vi "DAQ Process.vi"(10 "DAQ Process UE Refnum":T1, 11 "All Stop":refnum<user-event>) -> ()   [LabVIEW 2011]
doc: "Continuously generates Data and Error user events for the DAQ Process."
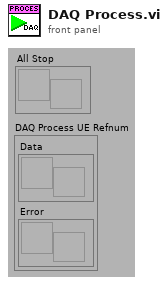
[diagram p1: front panel]
types:
  T1 = cluster{"Data":refnum<user-event>, "Error":refnum<user-event>}
  T2 = cluster{"seconds since 1Jan1904":timestamp, i32, dbl[]}
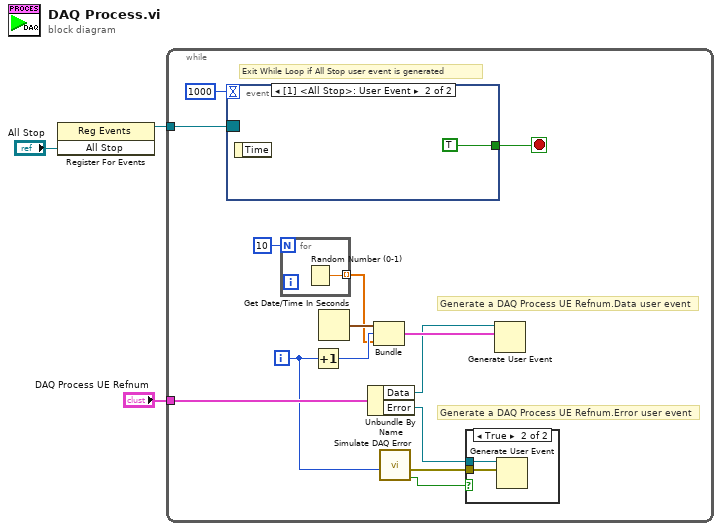
[diagram p0: block diagram]
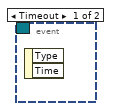
[diagram p3: hidden frame]
diagram:
  n1 = register-events("All Stop") -> (reference out=w2:refnum<event-registration>)  [unwired: 2 in, 1 out]
  n2 = while {
    tunnel: w2 -> [w15]
    tunnel: "DAQ Process UE Refnum" -> [w13]
    i -> [w8]
    stop <- w16 stop-if-true
    # "Generate a DAQ Process UE Refnum.Error user event"
    # "Generate a DAQ Process UE Refnum.Data user event"
    # "Exit While Loop if All Stop user event is generated"
    n3 = event shown="[1] <All Stop>: User Event" {
      selector: w15 -> [_ _]
      dyn-events: _ -> [_ _]
      timeout: 1000 -> [_ _]
      tunnel: [_ TRUE] -> w16
      event Timeout {
        n4 = event-data() -> ()  [unwired: 1 in, 2 out]
      }
      event User Event {
        n5 = event-data() -> ()  [unwired: 1 in, 1 out]
      }
    }
    n6 = for {
      N: 10 -> [_]
      tunnel: [w20] -> w10 mode=indexing
      n7 = Random Number (0-1)() -> (number: 0 to 1=w20:dbl)
    }
    n8 = Increment(x=w8) -> (x+1=w11:i32)
    n9 = Get Date/Time In Seconds() -> (seconds since 1Jan1904=w12:timestamp)
    n10 = Unbundle By Name(w13) -> ("Data"=w5:refnum<user-event>, "Error"=w6:refnum<user-event>)
    n11 = Bundle("seconds since 1Jan1904"=w12, w11, w10) -> (w9:T2)  [unwired: 1 in]
    n12 = call "Simulate DAQ Error.vi"("Iteration"=w8) -> ("Error?"=w4:bool, "error out"=w7:errorcluster)  [unwired: 9 in]
    n13 = case shown="True" w4 {
      tunnel: w7 -> [_ w19]
      tunnel: w6 -> [_ w18]
      frame False {
      }
      frame True {
        n14 = Generate User Event(user event=w18, event data cluster=w19) -> ()  [unwired: 1 in, 2 out]
      }
    }
    n15 = Generate User Event(user event=w5, event data cluster=w9) -> ()  [unwired: 1 in, 2 out]
  }
